vi "mod_MtoBitsperSymbol.vi"(1 "M":i32=2) -> (0 "Bits/ Symbol":i32)   [LabVIEW 2020, in "niDMT.lvlib"]
uses:
  <vilib>/addons/Modulation/niDMT.lvlib
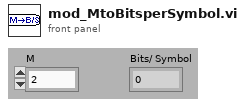
[diagram p1: front panel]
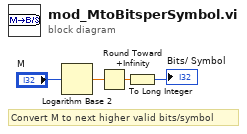
[diagram p0: block diagram]
diagram:
  # "Convert M to next higher valid bits/symbol"
  n1 = Logarithm Base 2(1:"M") -> (0:w2:dbl)
  n2 = Round Toward +Infinity(x=w2) -> (ceil(x): smallest int >= x=w3:dbl)
  n3 = To Long Integer(number=w3) -> (32bit integer=→"Bits/ Symbol":i32)
